vi "test_numberic_type_def.vi"() -> ()   [LabVIEW 2021]
uses:
  numeric_type_def.ctl
panel:
  in  "Numeric":T1 scale=0.0..10.0
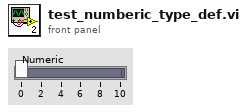
[diagram p1: front panel]
types:
  T1 = typedef "numeric_type_def.ctl" = dbl
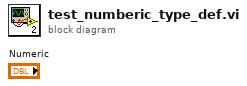
[diagram p0: block diagram]
diagram:
